vi "Intake level 2.vi"(9 "Left":T1={"DeviceStatus"={"status"=FALSE, "code"=0, "source"=""}, "Type"=enum."PWM", "PWM"={"PWM Channel"=enum."PWM 7", "DeadBand"={"Name"="Talon", "maxPositivePwm"=1537, "minPositivePwm"=1020, "centerPwm"=1013, "maxNegativePwm"=1006, "minNegativePwm"=489, "angularRange"=0}}, "CAN"={"Device Number"=0, "SetOutput VI Ref"=variant(refnum<vi> refnum), "GetOutput VI Ref"=variant(refnum<vi> refnum), "Enable VI Ref"=variant(refnum<vi> refnum), "Disable VI Ref"=variant(refnum<vi> refnum), "Data"=variant}, "Invert"=FALSE, "DIO PWM"={"PWM \"Enable\" Channel"=enum."Invalid", "DIOChannel"=enum."Invalid", "PWM Rate"=0.0}}, 10 "Right":T1={"DeviceStatus"={"status"=FALSE, "code"=0, "source"=""}, "Type"=enum."PWM", "PWM"={"PWM Channel"=enum."PWM 2", "DeadBand"={"Name"="Talon", "maxPositivePwm"=1537, "minPositivePwm"=1020, "centerPwm"=1013, "maxNegativePwm"=1006, "minNegativePwm"=489, "angularRange"=0}}, "CAN"={"Device Number"=0, "SetOutput VI Ref"=variant(refnum<vi> refnum), "GetOutput VI Ref"=variant(refnum<vi> refnum), "Enable VI Ref"=variant(refnum<vi> refnum), "Disable VI Ref"=variant(refnum<vi> refnum), "Data"=variant}, "Invert"=FALSE, "DIO PWM"={"PWM \"Enable\" Channel"=enum."Invalid", "DIOChannel"=enum."Invalid", "PWM Rate"=0.0}}) -> ()   [LabVIEW 2017]
uses:
  <vilib>/Rock Robotics/WPI/MotorControl/WPI_MotorControlDeviceRef.ctl
  <vilib>/Rock Robotics/WPI/MotorControl/WPI_MotorControlType.ctl
  <vilib>/Rock Robotics/SystemInterfaces/DIO/FPGA_DIOPWMChannel.ctl
  <vilib>/Rock Robotics/WPI/PWM/WPI_PWMDeadband.ctl
  <vilib>/Rock Robotics/SystemInterfaces/DIO/FPGA_DIOChannel.ctl
  <vilib>/Platform/TimedLoop/XDataNode/timing_clust.ctl
  <vilib>/Platform/TimedLoop/XDataNode/nitl_modes.ctl
  <vilib>/Platform/TimedLoop/XDataNode/wakeup.ctl
  <vilib>/Rock Robotics/WPI/DriverStation/WPI_DriverStationRobotMode2.ctl
  <userlib>/836-Library/System/TDMS_V2/Support/Logging_Settings.ctl
  <userlib>/836-Library/System/TDMS_V2/Support/Group_FIFO_Config.ctl
  <userlib>/836-Library/System/TDMS_V2/Support/Channel_FIFO_Config.ctl
  LevelOne/IntakeScore Enum.ctl
  CommandTypes/LiftCommands.ctl
  CommandTypes/DriveCommands.ctl
  CommandTypes/IntakeCommands.ctl
  <vilib>/platform/TimedLoop/XDataNode/XDataNode.xnode
  <vilib>/Platform/TimedLoop/XDataNode/XDNodeRunTimeDep.lvlib
panel:
  in  "Out Home Behind":dbl=1.0
  in  "Out Home":dbl=1.0
  in  "Out Ground Behind":dbl=1.0
  in  "Out Switch Behind":dbl=1.0
  in  "Out Low Behind":dbl=0.4
  in  "Out Med Behind":dbl=0.5
  in  "Out High Behind":dbl=0.6
  in  "Out Ground":dbl=1.0
  in  "Out Switch":dbl=0.5
  in  "Out Low":dbl=0.4
  in  "Out Med":dbl=0.45
  in  "Out High":dbl=0.45
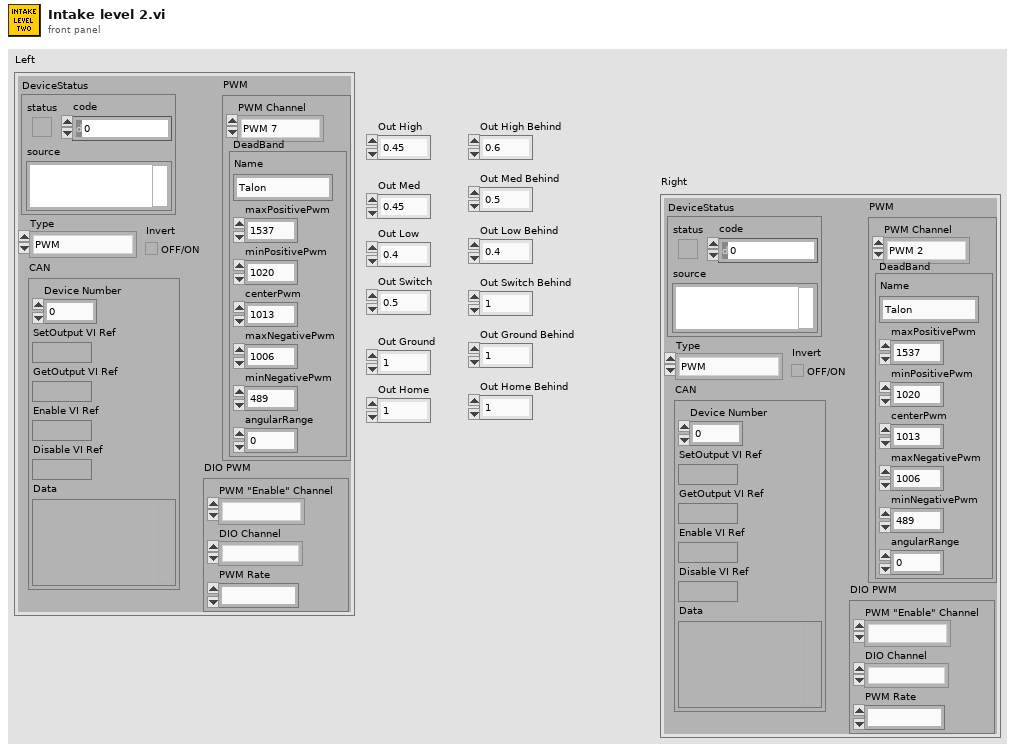
[diagram p1: front panel]
types:
  T1 = typedef "WPI_MotorControlDeviceRef.ctl" = cluster{"DeviceStatus":errorcluster, "Type":T2, "PWM":cluster{"PWM Channel":T3, "DeadBand":T4}, "CAN":cluster{"Device Number":u8, "SetOutput VI Ref":variant, "GetOutput VI Ref":variant, "Enable VI Ref":variant, "Disable VI Ref":variant, "Data":variant}, "Invert":bool, "DIO PWM":cluster{"PWM \"Enable\" Channel":T3, "DIOChannel":T5, "PWM Rate":dbl}}
  T2 = typedef "WPI_MotorControlType.ctl" = enum16{"PWM", "CAN", "DIO PWM"}
  T3 = typedef "FPGA_DIOPWMChannel.ctl" = enum8{"PWM 0", "PWM 1", "PWM 2", "PWM 3", "PWM 4", "PWM 5", "PWM 6", "PWM 7", "PWM 8", "PWM 9", "PWM MXP 0", "PWM MXP 1", "PWM MXP 2", "PWM MXP 3", "PWM MXP 4", "PWM MXP 5", "PWM MXP 6", "PWM MXP 7", "PWM MXP 8", "PWM MXP 9", "Invalid"}
  T4 = typedef "WPI_PWMDeadband.ctl" = cluster{"Name":string, "maxPositivePwm":i32, "minPositivePwm":i32, "centerPwm":i32, "maxNegativePwm":i32, "minNegativePwm":i32, "angularRange":u16}
  T5 = typedef "FPGA_DIOChannel.ctl" = enum8{"DIO 0", "DIO 1", "DIO 2", "DIO 3", "DIO 4", "DIO 5", "DIO 6", "DIO 7", "DIO 8", "DIO 9", "DIO MXP 0", "DIO MXP 1", "DIO MXP 2", "DIO MXP 3", "DIO MXP 4", "DIO MXP 5", "DIO MXP 6", "DIO MXP 7", "DIO MXP 8", "DIO MXP 9", "DIO MXP 10", "DIO MXP 11", "DIO MXP 12", "DIO MXP 13", "DIO MXP 14", "DIO MXP 15", "SPI Port CS1", "SPI Port CS2", "SPI Port CS3", "SPI Port MISO", "SPI Port MOSI", "Invalid"}
  T6 = typedef "XDNodeRunTimeDep.lvlib/timing_clust.ctl" = cluster{"Expected End [f-1]":u64, "Actual End [f-1]":u64, "Finished Late? [f-1]":bool, "Expected End [i-1]":u64, "Actual End [i-1]":u64, "Finished Late? [i-1]":bool, "Expected Start [i]":u64, "Actual Start [i]":u64, "Expected Start [f]":u64, "Actual Start [f]":u64, "Source Name":string, "Structure Name":string, "Period":i64, "Deadline":i64, "Offset":i64, "Start":i64, "Priority":i32, "Timeout":i32, "Mode":T7, "Wakeup Reason":T8, "Error":errorcluster, "Source Type":string, "Secondary Source Type":string, "Global End Time":u64, "Global Start Time":u64, "Frame Duration":u64, "Iteration Duration":u64, "Assigned CPU":i32, "I/O Scan Engine Mode":u32}
  T7 = typedef "XDNodeRunTimeDep.lvlib/nitl_modes.ctl" = enum32{"No Change", "Process missed periods, maintain original phase", "Discard missed periods, maintain original phase", "Process missed periods, ignore original phase", "Discard missed periods, ignore original phase"}
  T8 = typedef "XDNodeRunTimeDep.lvlib/wakeup.ctl" = enum32{"Normal", "Aborted", "Asynchronous wakeup", "Timing source error", "Timed loop error", "Timeout"}
  T9 = typedef "WPI_DriverStationRobotMode2.ctl" = enum16{"Autonomous Disabled", "Autonomous Enabled", "Teleop Disabled", "Teleop Enabled", "Disconnected", "Finish", "Test Disabled", "Test Enabled", "Emergency Stopped"}
  T10 = enum16{"Do Nothing", "Manuel", "Score", "Acquire"}
  T11 = typedef "IntakeScore Enum.ctl" = enum16{"Outake", "Intake", "Do nothing"}
  T12 = enum16{"Center on Cube", "Manual", "Acquire Cube", "Drive Path"}
  T13 = typedef "LiftCommands.ctl" = enum16{"Do  Nothing", "Manuel", "Ground", "Home", "To Switch", "To Scale Low", "To Scale Medium", "To Scale High", "Climb"}
  T14 = typedef "IntakeCommands.ctl" = enum16{"Do Nothing", "Manuel", "Score", "Acquire"}
  T15 = typedef "DriveCommands.ctl" = enum16{"Center on Cube", "Manual", "Acquire Cube", "Drive Path"}
  T16 = typedef "Logging_Settings.ctl" = cluster{"Data Grab Period":dbl, "File Write Period":dbl, "Max Stored Size":dbl, "Burst Size":dbl}
  T17 = typedef "Group_FIFO_Config.ctl" = cluster{"Group":string, "Channels":T18[], "Channel Names":string[]}
  T18 = typedef "Channel_FIFO_Config.ctl" = cluster{"Channel":string, "FIFO":refnum<k33>}
  T19 = typedef "Semaphore RefNum" = refnum<k1>
  T20 = cluster{"Name":string, "File Ref":refnum<k34>, "Start Time":timestamp, "Logging Settings":T16, "Group FIFO Config":T17[], "Data To Write":refnum<data-value>, "semaphore":T19}
  T21 = enum16{"Do  Nothing", "Manuel", "Ground", "Home", "To Switch", "To Scale Low", "To Scale Medium", "To Scale High", "Climb"}
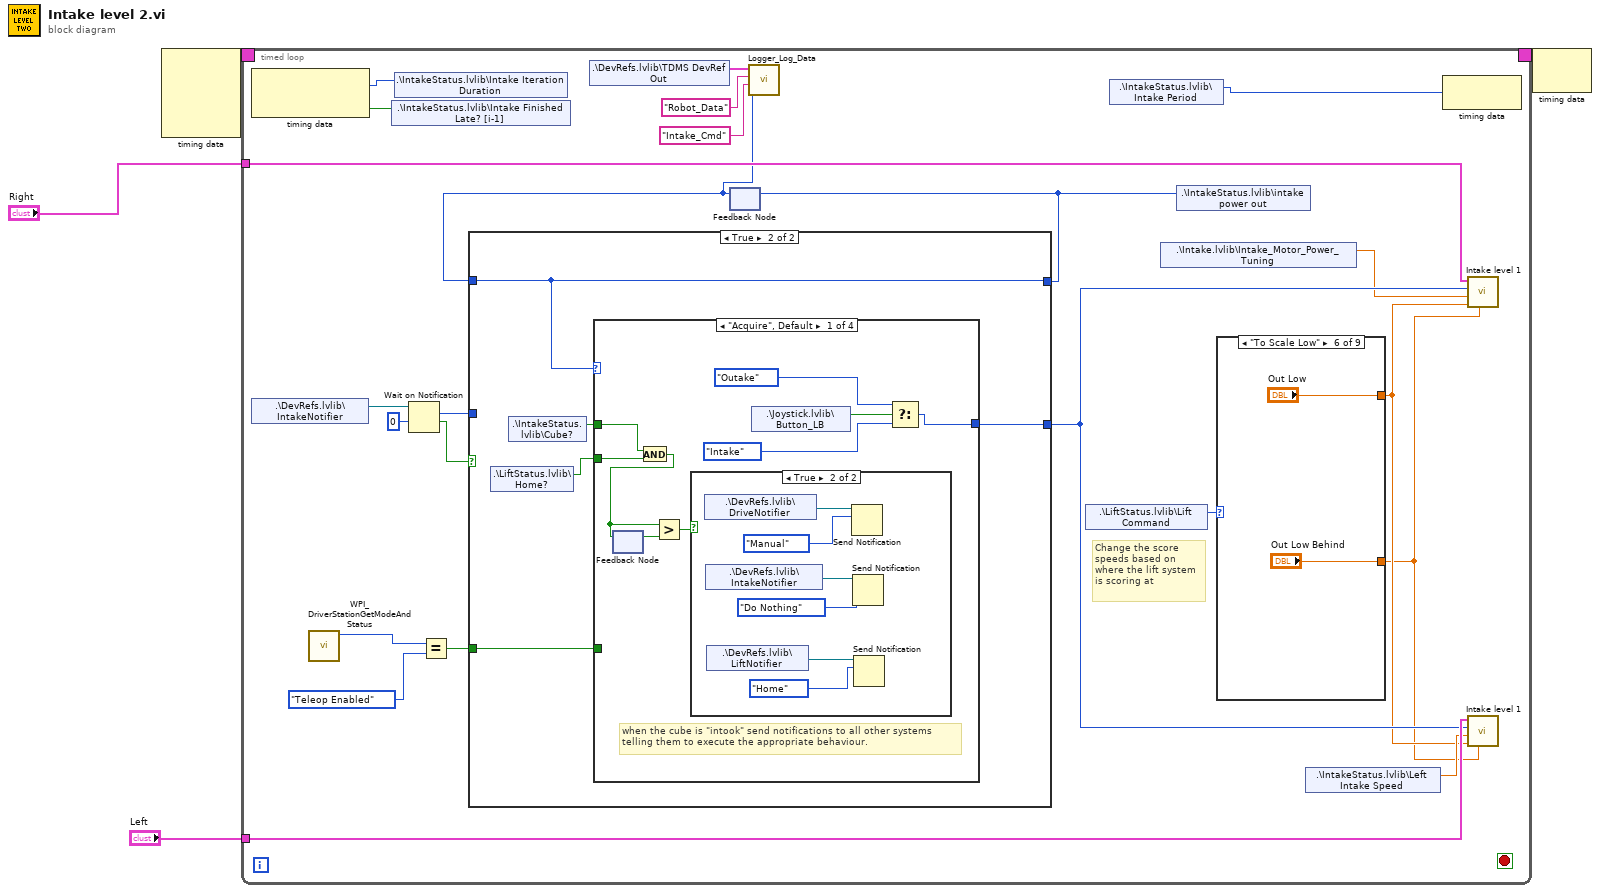
[diagram p0: block diagram]
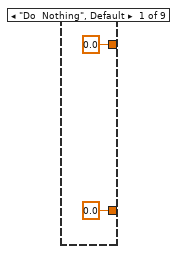
[diagram p2: hidden frame]
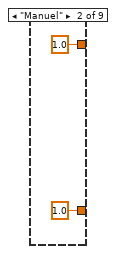
[diagram p3: hidden frame]
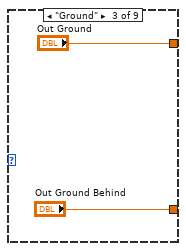
[diagram p4: hidden frame]
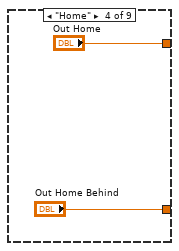
[diagram p5: hidden frame]
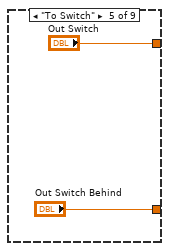
[diagram p6: hidden frame]
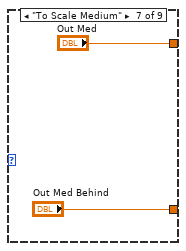
[diagram p7: hidden frame]
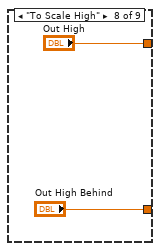
[diagram p8: hidden frame]
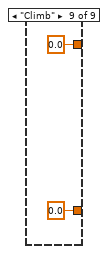
[diagram p9: hidden frame]
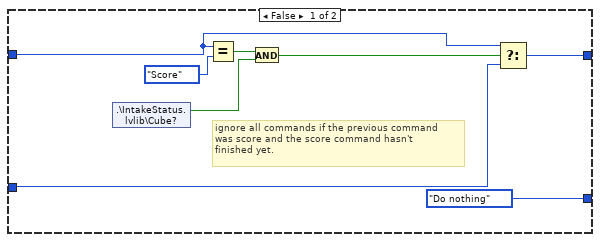
[diagram p10: hidden frame]
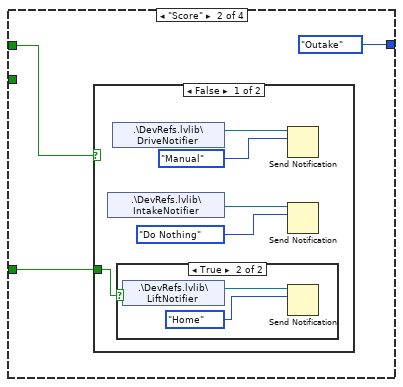
[diagram p12: hidden frame]
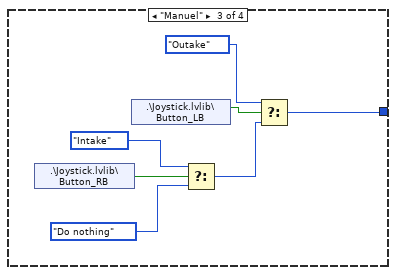
[diagram p15: hidden frame]
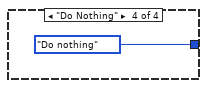
[diagram p16: hidden frame]
diagram:
  n1 = node-c288() -> (w4:T6)  [unwired: 4 in]
  n2 = timed-loop {
    timing: w4 -> [_]
    timing-out: [_] -> w3
    tunnel: "Right" -> [w27]
    tunnel: "Left" -> [w14]
    stop <- _ stop-if-true
    # "Change the score\nspeeds based on \nwhere the lift system\nis scoring at"
    n3 = node-c288() -> (w22:i64, w21:bool)  [unwired: 1 in]
    n4 = shared-variable ".\\DevRefs.lvlib\\IntakeNotifier"() -> (w26:refnum<notifier>)  [unwired: 1 in, 1 out]
    n5 = call <vilib>:"WPI_DriverStationGetModeAndStatus.vi"() -> ("Robot Mode"=w7:T9)  [unwired: 10 in, 1 out]
    n6 = shared-variable ".\\IntakeStatus.lvlib\\Intake Finished Late? [i-1]"(w21) -> ()  [unwired: 1 in, 1 out]
    n7 = shared-variable ".\\IntakeStatus.lvlib\\Intake Iteration Duration"(w22) -> ()  [unwired: 1 in, 1 out]
    n8 = Wait on Notification(notifier=w26, timeout in ms (-1)=0) -> (notification=w24:T10, timed out?=w25:bool)  [unwired: 2 in, 2 out]
    n9 = Equal?(x=w7, y=WPI_DriverStationRobotMode2."Teleop Enabled") -> (x = y?=w5:bool)
    n10 = shared-variable ".\\DevRefs.lvlib\\TDMS DevRef Out"() -> (w18:T20)  [unwired: 1 in, 1 out]
    n11 = feedback #1() -> (w15:T10)  [unwired: 1 in]
    n12 = case shown="True" w25 {
      tunnel: [IntakeScore_Enum."Do nothing" ("Command") w58] -> w13
      tunnel: w24 -> [w46 _]
      tunnel: [w52 w56] -> w19
      tunnel: w15 -> [w47 w56]
      tunnel: w5 -> [_ w54]
      frame False {
        # "ignore all commands if the previous command\nwas score and the score command hasn't\nfinished yet."
        n13 = shared-variable ".\\IntakeStatus.lvlib\\Cube?"() -> (w48:bool)  [unwired: 1 in, 1 out]
        n14 = Equal?(x=w47, y=T10."Score") -> (x = y?=w50:bool)
        n15 = And(x=w50, y=w48) -> (x .and. y?=w49:bool)
        n16 = Select(t=w47, s=w49, f=w46) -> (s? t:f=w52:T10)
      }
      frame True {
        n17 = shared-variable ".\\LiftStatus.lvlib\\Home?"() -> (w55:bool)  [unwired: 1 in, 1 out]
        n18 = shared-variable ".\\IntakeStatus.lvlib\\Cube?"() -> (w57:bool)  [unwired: 1 in, 1 out]
        n19 = case shown="\"Acquire\", Default" w56 {
          tunnel: [w64 IntakeScore_Enum."Outake" ("Command") w88 IntakeScore_Enum."Do nothing" ("Command")] -> w58
          tunnel: w57 -> [w61 w75 _ _]
          tunnel: w55 -> [w60 _ _ _]
          tunnel: w54 -> [_ w74 _ _]
          frame "Acquire", Default {
            # "when the cube is \"intook\" send notifications to all other systems\ntelling them to execute the appropriate behaviour."
            n20 = feedback #2() -> (w67:bool)  [unwired: 1 in]
            n21 = And(x=w61, y=w60) -> (x .and. y?=w59:bool)
            n22 = feedback-in #2(w59) -> ()
            n23 = Greater?(x=w59, y=w67) -> (0:w66:bool)
            n24 = case shown="True" w66 {
              frame False {
              }
              frame True {
                n25 = shared-variable ".\\DevRefs.lvlib\\DriveNotifier"() -> (w73:refnum<notifier>)  [unwired: 1 in, 1 out]
                n26 = shared-variable ".\\DevRefs.lvlib\\IntakeNotifier"() -> (w72:refnum<notifier>)  [unwired: 1 in, 1 out]
                n27 = shared-variable ".\\DevRefs.lvlib\\LiftNotifier"() -> (w71:refnum<notifier>)  [unwired: 1 in, 1 out]
                n28 = Send Notification(notification=T12."Manual", notifier=w73) -> ()  [unwired: 1 in, 2 out]
                n29 = Send Notification(notification=T10."Do Nothing", notifier=w72) -> ()  [unwired: 1 in, 2 out]
                n30 = Send Notification(notification=LiftCommands."Home", notifier=w71) -> ()  [unwired: 1 in, 2 out]
              }
            }
            n31 = shared-variable ".\\Joystick.lvlib\\Button_LB"() -> (w62:bool)  [unwired: 1 in, 1 out]
            n32 = Select(t=IntakeScore_Enum."Outake" ("Command"), s=w62, f=IntakeScore_Enum."Intake" ("Command")) -> (s? t:f=w64:T11)
          }
          frame "Score" {
            n33 = case shown="False" w75 {
              tunnel: w74 -> [w77 _]
              frame False {
                n34 = shared-variable ".\\DevRefs.lvlib\\IntakeNotifier"() -> (w79:refnum<notifier>)  [unwired: 1 in, 1 out]
                n35 = shared-variable ".\\DevRefs.lvlib\\DriveNotifier"() -> (w81:refnum<notifier>)  [unwired: 1 in, 1 out]
                n36 = case shown="True" w77 {
                  frame False {
                  }
                  frame True {
                    n37 = shared-variable ".\\DevRefs.lvlib\\LiftNotifier"() -> (w83:refnum<notifier>)  [unwired: 1 in, 1 out]
                    n38 = Send Notification(notification=LiftCommands."Home", notifier=w83) -> ()  [unwired: 1 in, 2 out]
                  }
                }
                n39 = Send Notification(notification=DriveCommands."Manual", notifier=w81) -> ()  [unwired: 1 in, 2 out]
                n40 = Send Notification(notification=IntakeCommands."Do Nothing", notifier=w79) -> ()  [unwired: 1 in, 2 out]
              }
              frame True {
              }
            }
          }
          frame "Manuel" {
            n41 = shared-variable ".\\Joystick.lvlib\\Button_RB"() -> (w85:bool)  [unwired: 1 in, 1 out]
            n42 = shared-variable ".\\Joystick.lvlib\\Button_LB"() -> (w84:bool)  [unwired: 1 in, 1 out]
            n43 = Select(t=IntakeScore_Enum."Intake" ("Command"), s=w85, f=IntakeScore_Enum."Do nothing" ("Command")) -> (s? t:f=w87:T11)
            n44 = Select(t=IntakeScore_Enum."Outake" ("Command"), s=w84, f=w87) -> (s? t:f=w88:T11)
          }
          frame "Do Nothing" {
          }
        }
      }
    }
    n45 = feedback-in #1(w19) -> ()
    n46 = call <userlib>:"Logger_Log_Data.vi"("Data"=w15, "Channel"="Intake_Cmd", "Group"="Robot_Data", "TDMS DevRef"=w18) -> ()  [unwired: 7 in, 1 out]
    n47 = shared-variable ".\\LiftStatus.lvlib\\Lift Command"() -> (w10:T21)  [unwired: 1 in, 1 out]
    n48 = shared-variable ".\\IntakeStatus.lvlib\\Intake Period"() -> (w20:i64)  [unwired: 1 in, 1 out]
    n49 = shared-variable ".\\Intake.lvlib\\Intake_Motor_Power_Tuning"() -> (w12:dbl)  [unwired: 1 in, 1 out]
    n50 = shared-variable ".\\IntakeStatus.lvlib\\intake power out"(w19) -> ()  [unwired: 1 in, 1 out]
    n51 = case shown="\"To Scale Low\"" w10 {
      tunnel: [0.0 ("Out High") 1.0 ("Out High") "Out Ground" "Out Home" "Out Switch" "Out Low" "Out Med" "Out High" 0.0 ("Out High")] -> w9
      tunnel: [0.0 ("Out High Behind") 1.0 ("Out High Behind") "Out Ground Behind" "Out Home Behind" "Out Switch Behind" "Out Low Behind" "Out Med Behind" "Out High Behind" 0.0 ("Out High Behind")] -> w8
      frame "Do  Nothing", Default {
      }
      frame "Manuel" {
      }
      frame "Ground" {
      }
      frame "Home" {
      }
      frame "To Switch" {
      }
      frame "To Scale Low" {
      }
      frame "To Scale Medium" {
      }
      frame "To Scale High" {
      }
      frame "Climb" {
      }
    }
    n52 = shared-variable ".\\IntakeStatus.lvlib\\Left Intake Speed"() -> (w11:dbl)  [unwired: 1 in, 1 out]
    n53 = node-c288(w20) -> ()  [unwired: 1 out]
    n54 = call "Intake level 1.vi"("Behind Back Out Speed"=w8, "Out Speed"=w9, "Intake_Motor_Power"=w12, "Command"=w13, "MotorControlDevRef"=w27) -> ()  [unwired: 6 in, 1 out]
    n55 = call "Intake level 1.vi"("Behind Back Out Speed"=w8, "Out Speed"=w9, "Intake_Motor_Power"=w11, "Command"=w13, "MotorControlDevRef"=w14) -> ()  [unwired: 6 in, 1 out]
  }
  n56 = node-c288(w3) -> ()  [unwired: 1 out]
